vi "tsdb_get_flexray_frame_properties_by_address_verbose.vi"(8 "error in (no error)":errorcluster caption="错误输入（无错误）", 10 "AAddr":string, 11 "path in":path) -> (0 "error out":errorcluster caption="错误输出", 1 "flexray_frame_properties_by_address":T1, 2 "function return":i32, 3 "path out":path)   [LabVIEW 2014]
doc: "Function introduction: Obtain flexray frame attribute information through address\nCall location\nInput parameter adder: Address\nADBIndex：\n Database index\nAECUIndes: ECU index\nAFrameIndex：\n Frame index\nAIsTx：\n TX AFRChannelMask: Channel Mask\nAFRBaseCycle：\n Basic cycle\nAFRCycleRepetition：\n Repetitive cycle\nAFRIsStartupFrame：\n Is it the starting frame\nAFRSlotId：slotId AFRCycleMask：\n Periodic mask\nASignalCount：\n Number of signals\nAName：\n Database Name\nAComment：\n notes\nReturn value 0: Successful execution\nOther values: Failed"
uses:
  Typedef/FlexRay/flexray_frame_properties_by_address.ctl
panel:
  out "AAddr 2":string
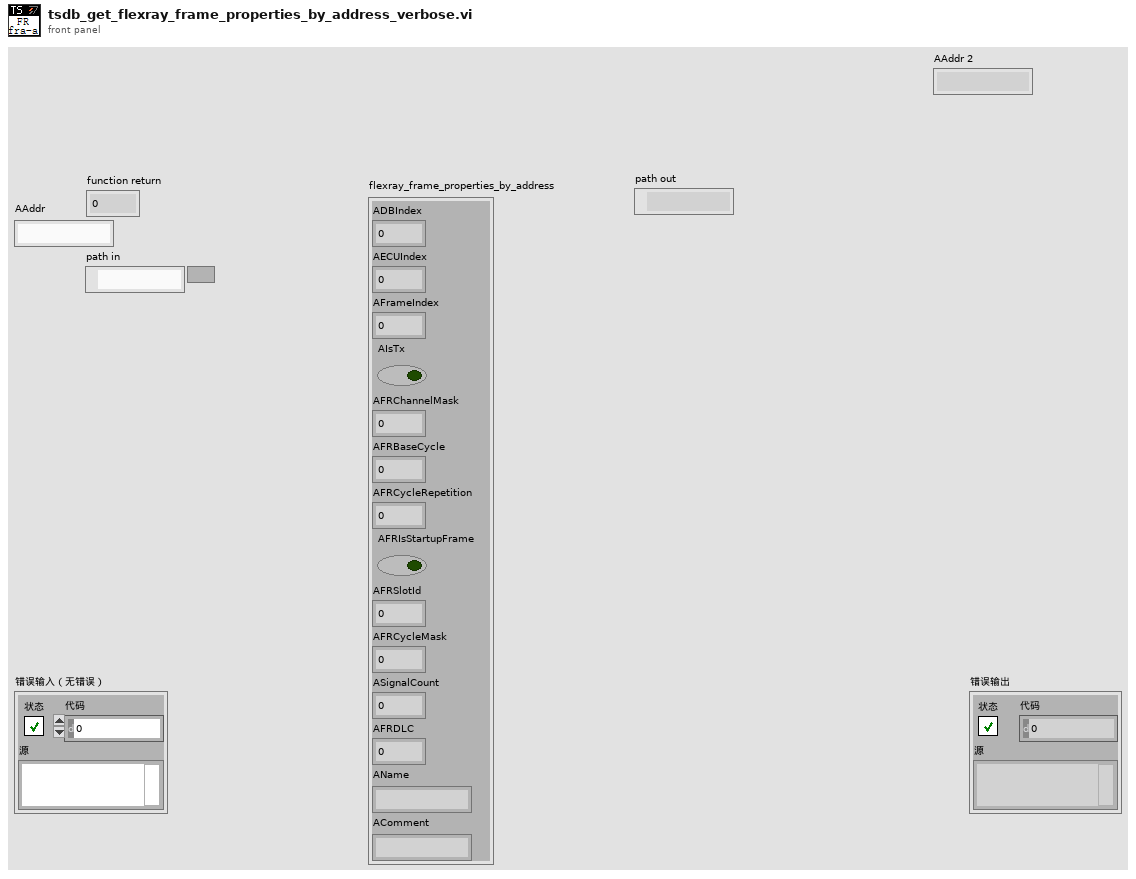
[diagram p1: front panel]
types:
  T1 = typedef "flexray_frame_properties_by_address.ctl" = cluster{"ADBIndex":i32, "AECUIndex":i32, "AFrameIndex":i32, "AIsTx":bool, "AFRChannelMask":i32, "AFRBaseCycle":i32, "AFRCycleRepetition":i32, "AFRIsStartupFrame":bool, "AFRSlotId":i32, "AFRCycleMask":i64, "ASignalCount":i32, "AFRDLC":i32, "AName":string, "AComment":string}
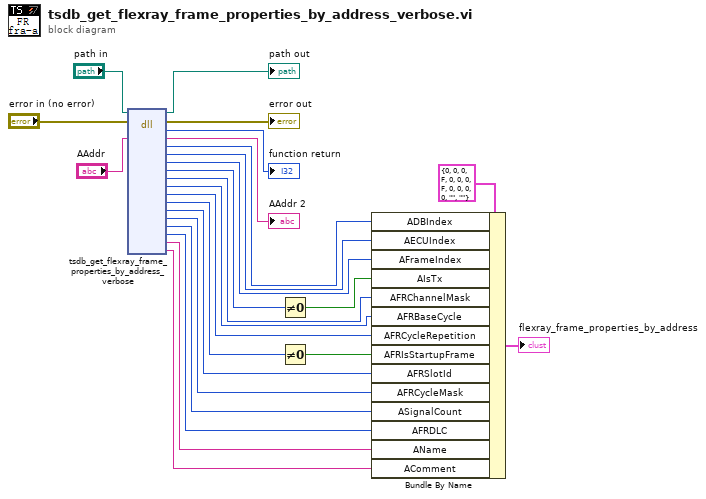
[diagram p0: block diagram]
diagram:
  n1 = dll-call lib="D:/Work/LabVIEW Code/TSMaster Labview SDK/LabVIEW/LabVIEW-TSMasterAPI_CLN/TSMasterAPI_LabVIEW-2024-10-08 14-20-13/Not_organized_vi/TSMaster.*" fn="tsdb_get_flexray_frame_properties_by_address_verbose"(path in="path in", error in="error in (no error)", "AAddr"="AAddr") -> (path out=→"path out":path, error out=→"error out":errorcluster, "返回类型"=→"function return":i32, "AAddr"=→"AAddr 2":string, "ADBIndex"=w12:i32, "AECUIndex"=w11:i32, "AFrameIndex"=w10:i32, "AIsTx"=w24:u8, "AFRChannelMask"=w9:i32, "AFRBaseCycle"=w8:i32, "AFRCycleRepetition"=w7:i32, "AFRIsStartupFrame"=w23:u8, "AFRSlotId"=w6:i32, "AFRCycleMask"=w5:i64, "ASignalCount"=w4:i32, "AFRDLC"=w3:i32, "AName"=w2:string, "AComment"=w1:string)  [unwired: 15 in]
  n2 = Not Equal To 0?(x=w24) -> (x != 0?=w14:bool)
  n3 = Not Equal To 0?(x=w23) -> (x != 0?=w13:bool)
  n4 = Bundle By Name(cluster=T1 {"ADBIndex"=0, "AECUIndex"=0, "AFrameIndex"=0, "AIsTx"=FALSE, "AFRChannelMask"=0, "AFRBaseCycle"=0, "AFRCycleRepetition"=0, "AFRIsStartupFrame"=FALSE, "AFRSlotId"=0, "AFRCycleMask"=0, "ASignalCount"=0, "AFRDLC"=0, "AName"="", "AComment"=""} ("flexray_frame_properties_by_address"), "ADBIndex"=w12, "AECUIndex"=w11, "AFrameIndex"=w10, "AIsTx"=w14, "AFRChannelMask"=w9, "AFRBaseCycle"=w8, "AFRCycleRepetition"=w7, "AFRIsStartupFrame"=w13, "AFRSlotId"=w6, "AFRCycleMask"=w5, "ASignalCount"=w4, "AFRDLC"=w3, "AName"=w2, "AComment"=w1) -> (→"flexray_frame_properties_by_address":T1)
